vi "430_RS232_Open.vi"(0 "VISA resource name":refnum<visa-resource-name>="COM1", 3 "timeout ms (2000)":i32=2000, 5 "error in (no error)":errorcluster) -> (6 "VISA resource name out":refnum<visa-resource-name>="COM1", 8 "error out":errorcluster)   [LabVIEW 2017]
uses:
  <vilib>/Instr/_visa.llb/VISA Configure Serial Port (Serial Instr).vi
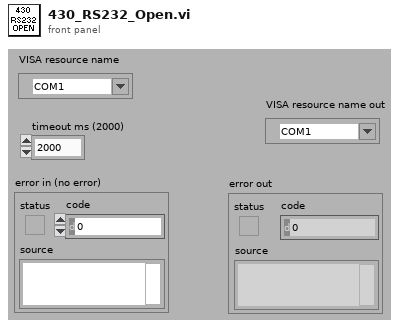
[diagram p1: front panel]
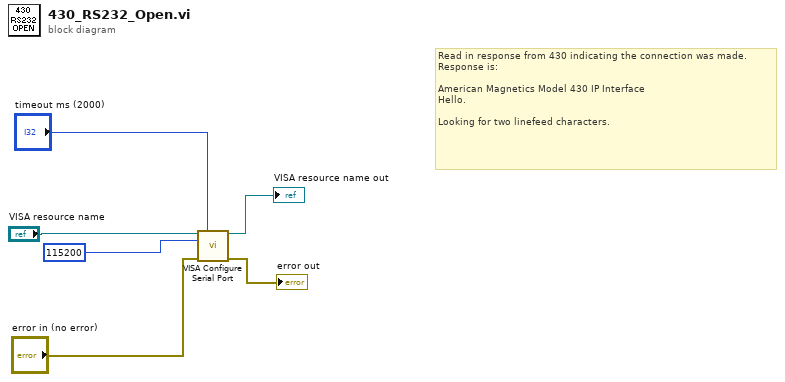
[diagram p0: block diagram]
diagram:
  # "Read in response from 430 indicating the connection was made.\nResponse is:\n\nAmerican Magnetics Model 430 IP Interface\nHello.\n\nLooking for two linefeed characters."
  n1 = call-poly "VISA Configure Serial Port"("VISA resource name"="VISA resource name", "timeout (10sec)"="timeout ms (2000)", "baud rate (9600)"=115200, "error in (no error)"="error in (no error)") -> ("VISA resource name out"=→"VISA resource name out":refnum<visa-resource-name>, "error out"=→"error out":errorcluster)  [unwired: 10 in]
